vi "Initialise Grid.vi"(8 "error in (no error)":errorcluster, 10 "Selection Grid":T1) -> (0 "error out":errorcluster, 1 "Valid":bool, 3 "Grassfire Algorithm out":refnum<class "Grassfire Algorithm.lvclass">)   [LabVIEW 2019, in "Grassfire Algorithm.lvclass"]
doc: "If a picture ring array is not used, use the following values:\n\n0 = free space\n1 = blocked\n2 = start point\n3 = end point"
uses:
  Grassfire Algorithm.lvclass
  Selection Grid Cell--array.ctl
  Selection--picture ring.ctl
  Grassfire Algorithm.lvclass/Grassfire Algorithm.ctl
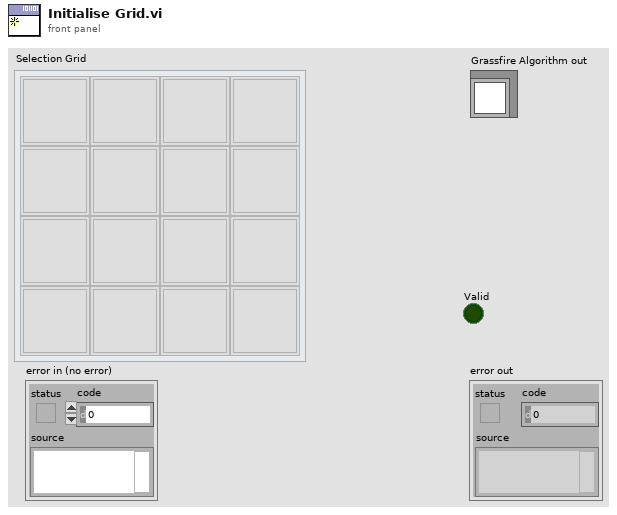
[diagram p1: front panel]
types:
  T1 = typedef "Grassfire Algorithm.lvclass/Selection Grid Cell--array.ctl" = cluster{"Grid Value":T2}[][]
  T2 = typedef "Grassfire Algorithm.lvclass/Selection--picture ring.ctl" = i64
  T3 = typedef "Grassfire Algorithm.lvclass/Grid Summary--cluster.ctl" = cluster{"Start":T4, "End":T4, "# Starts":i32, "# Empty":i32, "# Blocked":i32, "# End":i32}
  T4 = typedef "Grassfire Algorithm.lvclass/Index Column Row--cluster.ctl" = cluster{"Row":i32, "Column":i32}
  T5 = typedef "Grassfire Algorithm.lvclass/Solution Grid Cell Private--cluster.ctl" = cluster{"Picture":T6, "Value":dbl}
  T6 = typedef "Grassfire Algorithm.lvclass/Solution--picture ring.ctl" = i64
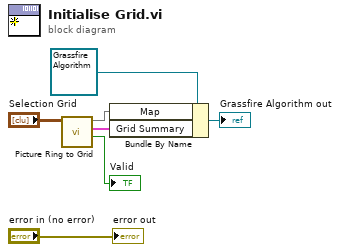
[diagram p0: block diagram]
diagram:
  n1 = call "Picture Ring to Grid.vi"("Selection Grid"="Selection Grid") -> ("Valid"=→"Valid":bool, "Grid Summary"=w3:T3, "Map"=w1:map{T4, T5})  [unwired: 8 in]
  n2 = Bundle By Name(cluster=refnum<class "Grassfire Algorithm.lvclass"> refnum ("Grassfire Algorithm in"), "Map"=w1, "Grid Summary"=w3) -> (→"Grassfire Algorithm out":refnum<class "Grassfire Algorithm.lvclass">)
  "error out" <- "error in (no error)"
